vi "receive error messages.vi"(9 "Queues":T1, 11 "comms in":T2) -> (3 "comms out":T2)   [LabVIEW 2018]
uses:
  type defs/comms loop data.ctl
  Chris VIs/Incident logger/Incident logger.lvclass
  type defs/Queues.ctl
  RT/Type Defs/generic incident.ctl
  <resource>/objmgr/ni.dex.rc
types:
  T1 = typedef "Queues.ctl" = cluster{"messageHandler":refnum<queue>, "comms":refnum<queue>, "dataStream":refnum<queue>, "dataProcessor":refnum<queue>, "fileIO":refnum<queue>, "userInterface":refnum<queue>, "errors":refnum<queue>, "customCompressor":refnum<queue>}
  T2 = typedef "comms loop data.ctl" = cluster{"params":cluster{"commandStream":cluster{"reader name":string, "RT IP address":string, "writer name":string, "stream buffer size":i32}, "errorStream":cluster{"reader name":string, "RT IP address":string, "writer name":string, "stream buffer size":i32}}, "vars":cluster{"errorStream":refnum<k21>, "commandStream":refnum<k21>, "Incident logger":refnum<class "Incident logger.lvclass">, "check error scheduled message":u32}}
  T3 = typedef "generic incident.ctl" = cluster{"timestamp":timestamp, "type":string, "Variant":variant}
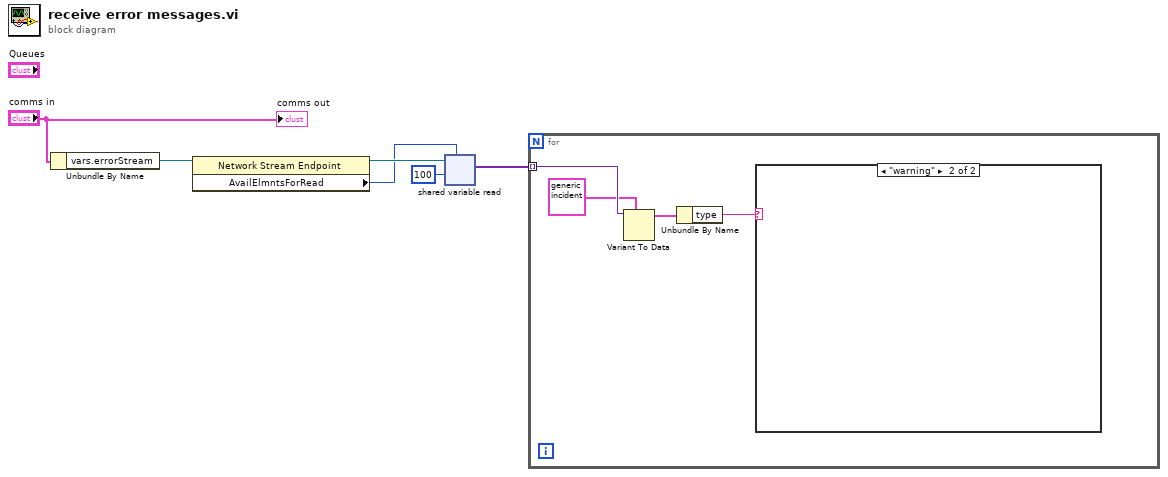
[diagram p0: block diagram]
diagram:
  n1 = Unbundle By Name("comms in") -> ("vars.errorStream"=w5:refnum<k21>)
  n2 = property class="Network Stream Endpoint"(reference=w5) -> (reference out=w4:refnum<k21>, "AvailElmntsForRead"=w3:i32)  [unwired: 1 in, 1 out]
  n3 = shared-variable-read(w4, 100 ("timeout ms (-1)"), w3) -> (w1:variant[])  [unwired: 1 in, 3 out]
  n4 = for {
    tunnel: w1 -> [w10] mode=indexing
    n5 = Variant To Data(type=T3 {"timestamp"=timestamp(0 s since 1904-01-01), "type"="", "Variant"=variant} ("incident cluster"), Variant=w10) -> (data=w8:T3)  [unwired: 1 in, 1 out]
    n6 = Unbundle By Name(w8) -> ("type"=w7:string)
    n7 = case shown="\"warning\"" w7 {
      frame "\u0000", Default {
      }
      frame "warning" {
      }
    }
  }
  "comms out" <- "comms in"
